vi "Create File.vi"() -> (0 "error out":errorcluster, 1 "Custom Device Name out":string, 3 "XML Path":path, 4 "Cancelled?":bool=TRUE)   [LabVIEW 2025]
uses:
  Types/XML Format String.ctl
panel:
  in  "Namespace Name":string="NationalInstruments.Veristand"
  in  "Custom Namespace Name":bool
  in  "Cancel":bool
  in  "Create":bool
  in  "Custom Device Name":string
  in  "XML Folder Path":path
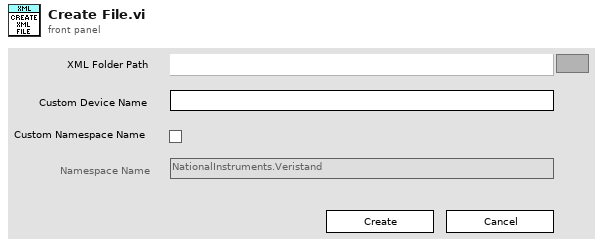
[diagram p1: front panel]
types:
  T1 = typedef "XML Format String.ctl" = string
  T2 = enum8{"Enabled", "Disabled", "Disabled and Grayed Out"}
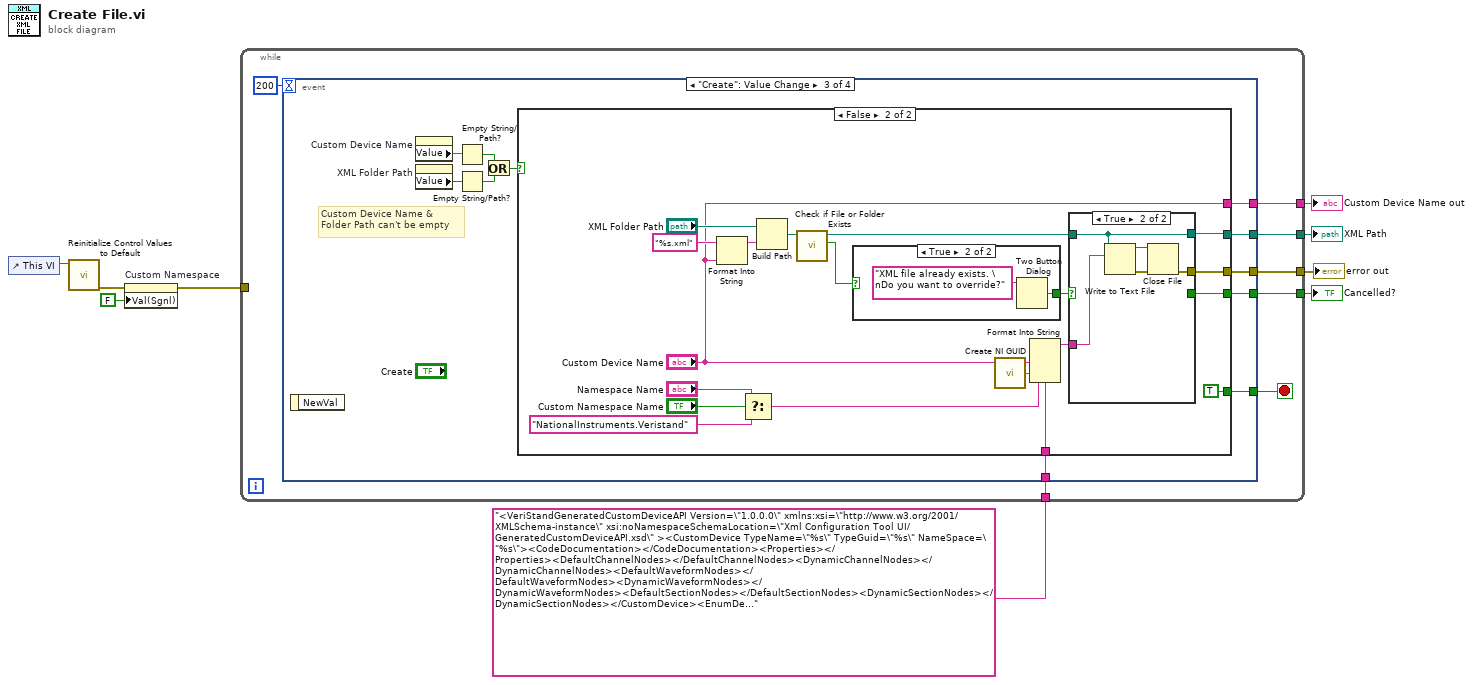
[diagram p0: block diagram]
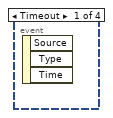
[diagram p2: hidden frame]
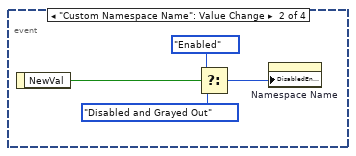
[diagram p3: hidden frame]
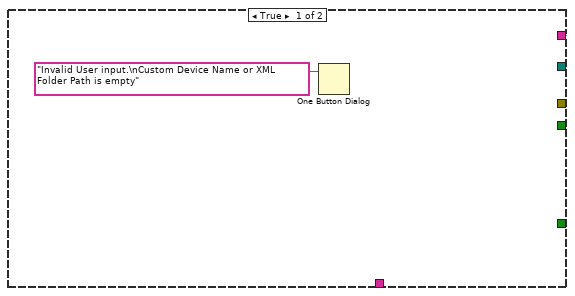
[diagram p4: hidden frame]
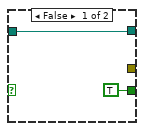
[diagram p5: hidden frame]
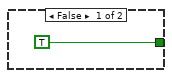
[diagram p6: hidden frame]
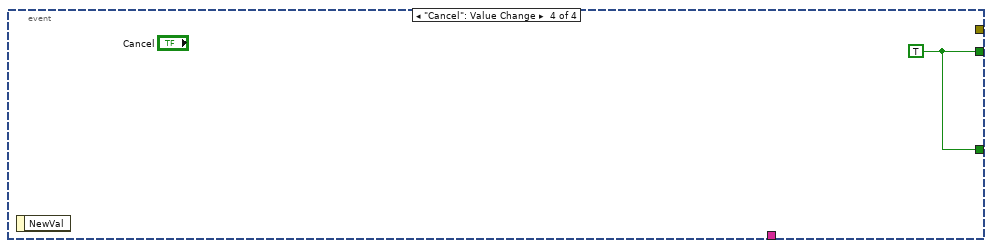
[diagram p7: hidden frame]
diagram:
  n1 = control-ref of="This VI"() -> (w5:refnum<vi>)
  n2 = call "Reinitialize Control Values to Default.vi"("VI Ref"=w5) -> ("error out"=w4:errorcluster)  [unwired: 10 in]
  n3 = property on="Custom Namespace" class="Bool (strict)"(error in=w4, "Val(Sgnl)"=FALSE ("Value (Signaling)")) -> (error out=w2:errorcluster)  [unwired: 1 in, 1 out]
  n4 = while {
    tunnel: [w15] -> w9
    tunnel: [w14] -> w8
    tunnel: [w13] -> w6
    tunnel: [w11] -> w7
    tunnel: w2 -> [_]
    tunnel: T1 "<VeriStandGeneratedCustomDeviceAPI Version=\"1.0.0.0\" xmlns:xsi=\"http://www.w3.org/2001/XMLSchema-instance\" xsi:noNamespaceSchemaLocation=\"Xml Configuration Tool UI/GeneratedCustomDeviceAPI.xsd\" ><CustomDevice TypeName=\"%s\" TypeGuid=\"%s\" NameSpace=\"%s\"><CodeDocumentation></CodeDocumentation><Properties></Properties><DefaultChannelNodes></DefaultChannelNodes><DynamicChannelNodes></DynamicChannelNodes><DefaultWaveformNodes></DefaultWaveformNodes><DynamicWaveformNodes></DynamicWaveformNodes><DefaultSectionNodes></DefaultSectionNodes><DynamicSectionNodes></DynamicSectionNodes></CustomDevice><EnumDefinitions></EnumDefinitions></VeriStandGeneratedCustomDeviceAPI>" ("XML Format") -> [w10]
    stop <- w16 stop-if-true
    n5 = event shown="[2] \"Create\": Value Change" {
      selector: _ -> [_ _ _ _]
      dyn-events: _ -> [_ _ _ _]
      timeout: 200 -> [_ _ _ _]
      tunnel: [_ _ w22 w63] -> w16
      tunnel: [_ _ w30 _] -> w15
      tunnel: [_ _ w29 _] -> w14
      tunnel: [_ _ w24 _] -> w13
      tunnel: [_ _ w23 w63] -> w11
      tunnel: w10 -> [_ _ w21 _]
      event Timeout {
        n6 = event-data() -> ()  [unwired: 1 in, 3 out]
      }
      event "Custom Namespace Name": Value Change {
        n7 = event-data() -> ("NewVal"=w20:bool)  [unwired: 1 in]
        n8 = Select(t=T2."Enabled" ("Disabled"), s=w20, f=T2."Disabled and Grayed Out" ("Disabled")) -> (s? t:f=w17:T2)
        n9 = property on="Namespace Name" class="Str"("DisabledEnum"=w17) -> ()  [unwired: 2 in, 2 out]
      }
      event "Create": Value Change {
        # "Custom Device Name &\nFolder Path can't be empty"
        n10 = event-data() -> ()  [unwired: 1 in, 1 out]
        n11 = property on="Custom Device Name" class="Str"() -> ("Value"=w31:string)  [unwired: 2 in, 2 out]
        n12 = property on="XML Folder Path" class="Path"() -> ("Value"=w28:path)  [unwired: 2 in, 2 out]
        n13 = Empty String/Path?(string/path=w31) -> (empty?=w26:bool)
        n14 = Empty String/Path?(string/path=w28) -> (empty?=w27:bool)
        n15 = Or(x=w26, y=w27) -> (x .or. y?=w25:bool)
        n16 = case shown="False" w25 {
          tunnel: ["" ("Value") "Custom Device Name"] -> w30
          tunnel: [_ w37] -> w29
          tunnel: [_ w48] -> w24
          tunnel: [_ w36] -> w23
          tunnel: [_ TRUE ("NewVal")] -> w22
          tunnel: w21 -> [_ w34]
          frame True {
            (unwired) "Custom Device Name or Namespace cannot be empty." ("Errors")
            n17 = One Button Dialog(message="Invalid User input.\nCustom Device Name or XML Folder Path is empty") -> ()  [unwired: 1 in, 1 out]
          }
          frame False {
            n18 = Format Into String(format string="%s.xml", "Custom Device Name") -> (resulting string=w51:string)  [unwired: 2 in, 1 out]
            n19 = Select(t="Namespace Name", s="Custom Namespace Name", f="NationalInstruments.Veristand" ("format string")) -> (s? t:f=w42:string)
            n20 = Build Path(base path="XML Folder Path", name or relative path=w51) -> (appended path=w41:path)
            n21 = call <vilib>:"Check if File or Folder Exists.vi"("path"=w41) -> ("file or folder exists?"=w39:bool, "dup path"=w40:path)  [unwired: 8 in, 1 out]
            n22 = case shown="True" w39 {
              tunnel: [TRUE ("T button?") w61] -> w38
              frame False {
              }
              frame True {
                n23 = Two Button Dialog(message="XML file already exists. \nDo you want to override?") -> (T button?=w61:bool)  [unwired: 2 in]
              }
            }
            n24 = call <vilib>:"Create NI GUID.vi"() -> ("NI GUID"=w50:string)
            n25 = Format Into String(format string=w34, "Custom Device Name", w50, w42) -> (resulting string=w52:string)  [unwired: 2 in, 1 out]
            n26 = case shown="True" w38 {
              tunnel: w52 -> [_ w59]
              tunnel: [_ w56] -> w48
              tunnel: w40 -> [w54 w55]
              tunnel: [w54 w55] -> w37
              tunnel: [TRUE _] -> w36
              frame False {
              }
              frame True {
                n27 = Write to Text File(file (use dialog)=w55, text=w59) -> (refnum out=w58:refnum<file>, error out=w57:errorcluster)  [unwired: 2 in, 1 out]
                n28 = Close File(refnum=w58, error in=w57) -> (error out=w56:errorcluster)  [unwired: 1 out]
              }
            }
          }
        }
      }
      event "Cancel": Value Change {
        w63 = TRUE ("NewVal")
        n29 = event-data() -> ()  [unwired: 1 in, 1 out]
      }
    }
  }
  "Custom Device Name out" <- w9
  "XML Path" <- w8
  "Cancelled?" <- w7
  "error out" <- w6
